vi "FPGA SPI_SPI Port.vi"(10 "Port":i8, 11 "FPGA IO":T1={"SCLK"="SCLK", "CS"="CS1", "MOSI"="MOSI", "MISO"="MISO"}) -> ()   [LabVIEW 2014]
uses:
  Controls/Port Action.ctl
  Controls/FPGA SPI_SPI Loop State.ctl
  <vilib>/Platform/TimedLoop/XDataNode/timing_clust.ctl
  <vilib>/Platform/TimedLoop/XDataNode/nitl_modes.ctl
  <vilib>/Platform/TimedLoop/XDataNode/wakeup.ctl
  <vilib>/rvi/Emulation/niFpgaGetClockAttributes.vi
  <vilib>/rvi/Emulation/niFpgaSctlEmulationGetInTimedLoop.vi
  <vilib>/rvi/Emulation/niFpgaEmulationReportErrorSimple.vi
  FPGA SPI_Globals.vi
  <vilib>/rvi/Emulation/niFpgaProcessEmulError.vi
  <vilib>/rvi/Emulation/niFpgaEmulationIsFPGAContextNoSignature.vi
  <vilib>/rvi/errors/niFpgaSetErrorForExecOnDevCompSimple.vi
  <vilib>/rvi/eio/common/nirviEmuReportErrorAndStop.vi
  <vilib>/rvi/DataTransferAndStorage/Container/Common/niFpgaContainerGetUniqueNameForEmu.vi
  <vilib>/rvi/FIFO/Fifo_Resource/nirvififoEmulationSetSize.vi
  <vilib>/rvi/FIFO/Fifo_Resource/nirviFifoEmulationQueueMgr.vi
  <instcachedir>/0/nirviFifoEmulationQueueMgr_E5CAEC123FF24DC58D834DCA3CDAA9B5.lvgen/nirviFifoEmulationQueueMgr_E5CAEC123FF24DC58D834DCA3CDAA9B5_001.vi
  <vilib>/rvi/FIFO/Fifo_Resource/nirvififoEmulationCreateLock.vi
  <vilib>/rvi/FIFO/Fifo_Resource/nirvififoEmulationObtainLock.vi
  <vilib>/rvi/FIFO/Fifo_Resource/nirvififoEmulationReleaseLock.vi
  <vilib>/rvi/occurrence/nirviWaitOnOccurrenceBase.vi
  <vilib>/rvi/errors/nirviReportUnexpectedCaseInternalError.vi
  <vilib>/rvi/errors/nirviReportUnexpectedCaseInternalError (U32).vi
  <vilib>/rvi/FIFO/Fifo_Resource/nirvififoEmulationDetermineInputValidOut.vi
  <vilib>/rvi/Emulation/niFpgaCriticalErrorInLSC.vi
  <vilib>/rvi/eio/common/nirviEmuTemplateMethod_errors.vi
  <vilib>/rvi/DataTransferAndStorage/Container/Common/niFpgaContainerSetEmuInfo.vi
  <vilib>/rvi/DataTransferAndStorage/Container/XNode/niFpgaContainer.xnode
  <vilib>/rvi/FIFO/Fifo_Resource/nirvififoEmulationRead.vi
  <vilib>/rvi/FIFO/Fifo_Resource/nirvififoEmulationWrite.vi
  <vilib>/Platform/TimedLoop/XDataNode/XDataNode.xnode
  <vilib>/eio/EIONode/EIONode.xnode
  <vilib>/rvi/LocalResourceManager/LocalResourceManager.xnode
  <vilib>/Platform/TimedLoop/XDataNode/XDNodeRunTimeDep.lvlib
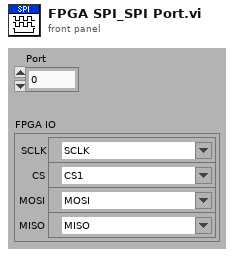
[diagram p1: front panel]
types:
  T1 = cluster{"SCLK":refnum<k21>, "CS":refnum<k21>, "MOSI":refnum<k21>, "MISO":refnum<k21>}
  T2 = cluster{"CS":u8, "CS Active State":bool, "CPOL":bool, "CPHA":bool, "Wait Ticks":u32}
  T3 = typedef "Port Action.ctl" = enum8{"Idle", "Start", "Configure Hardware", "Start Hardware", "Set Done", "Wait Until Done"}
  T4 = typedef "FPGA SPI_SPI Loop State.ctl" = enum8{"Initialize", "Read From FIFO", "Set CS", "Wait Before Set", "Set Clock", "Wait Before Reset", "Reset Clock", "Write to FIFO", "Reset CS"}
  T5 = typedef "XDNodeRunTimeDep.lvlib/timing_clust.ctl" = cluster{"Expected End [f-1]":u64, "Actual End [f-1]":u64, "Finished Late? [f-1]":bool, "Expected End [i-1]":u64, "Actual End [i-1]":u64, "Finished Late? [i-1]":bool, "Expected Start [i]":u64, "Actual Start [i]":u64, "Expected Start [f]":u64, "Actual Start [f]":u64, "Source Name":string, "Structure Name":string, "Period":i64, "Deadline":i64, "Offset":i64, "Start":i64, "Priority":i32, "Timeout":i32, "Mode":T6, "Wakeup Reason":T7, "Error":errorcluster, "Source Type":string, "Secondary Source Type":string, "Global End Time":u64, "Global Start Time":u64, "Frame Duration":u64, "Iteration Duration":u64, "Assigned CPU":i32, "I/O Scan Engine Mode":u32}
  T6 = typedef "XDNodeRunTimeDep.lvlib/nitl_modes.ctl" = enum32{"No Change", "Process missed periods, maintain original phase", "Discard missed periods, maintain original phase", "Process missed periods, ignore original phase", "Discard missed periods, ignore original phase"}
  T7 = typedef "XDNodeRunTimeDep.lvlib/wakeup.ctl" = enum32{"Normal", "Aborted", "Asynchronous wakeup", "Timing source error", "Timed loop error", "Timeout"}
  T8 = typedef "FPGA SPI_FPGA SPI State.ctl" = enum8{"Idle", "Read/Write SPI", "Configure"}
  T9 = cluster{"MOSI":bool[], "MISO":bool[], "MOSI Byte Index":i8, "MISO Byte Index":i8}
  T10 = cluster{"Next State":T4, "Wait Count":u32, "Total Bits":u16, "Current Bit":u16, "Total Bytes":u16}
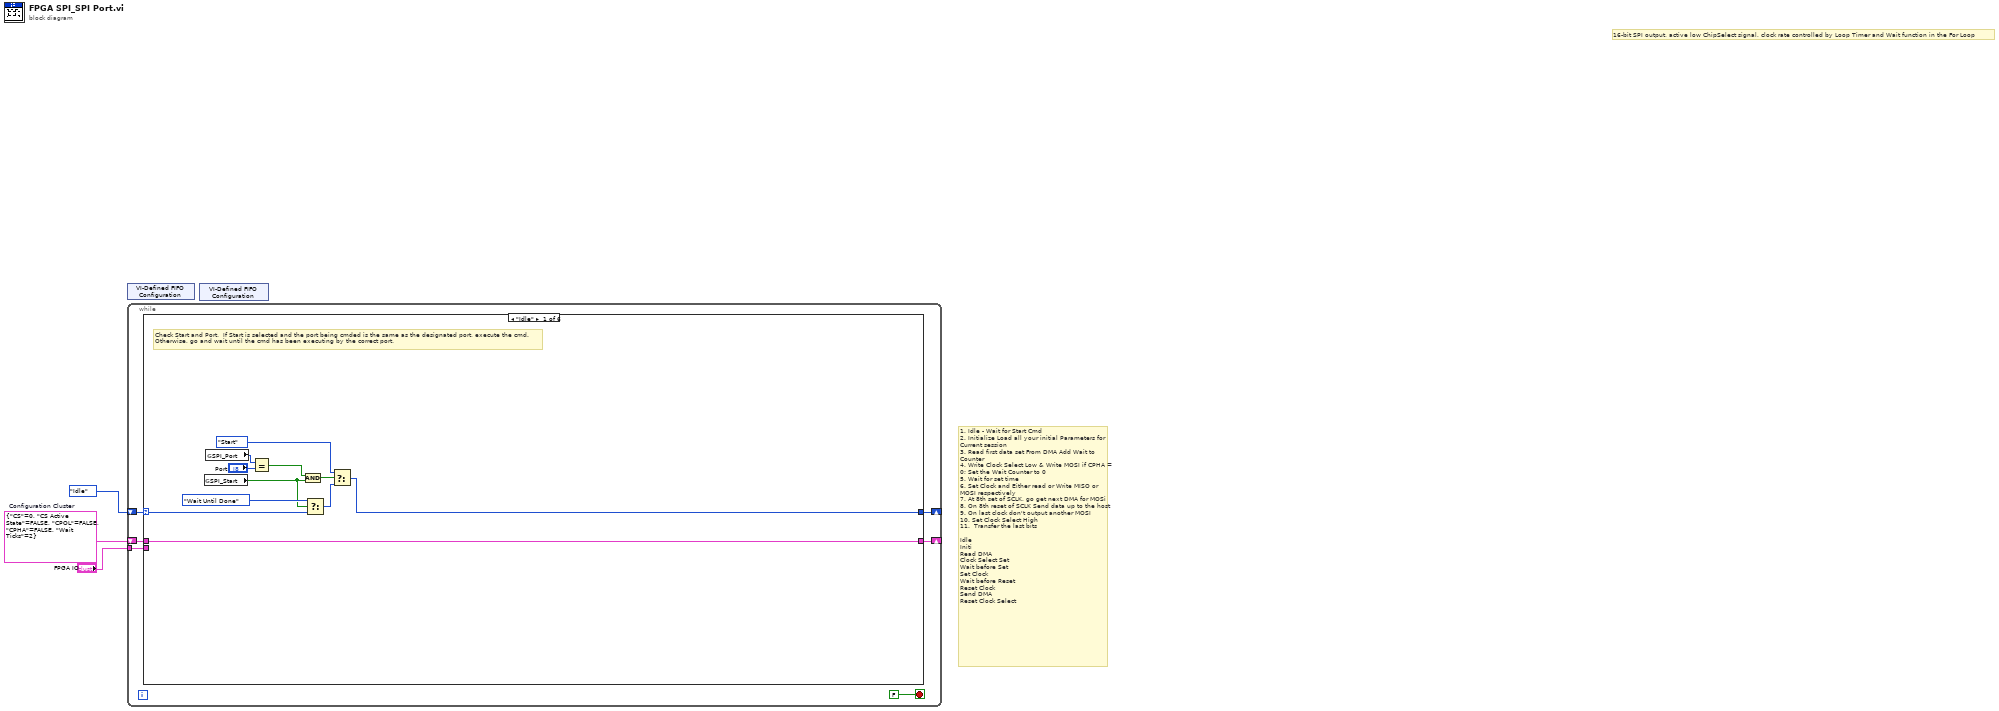
[diagram p0: block diagram]
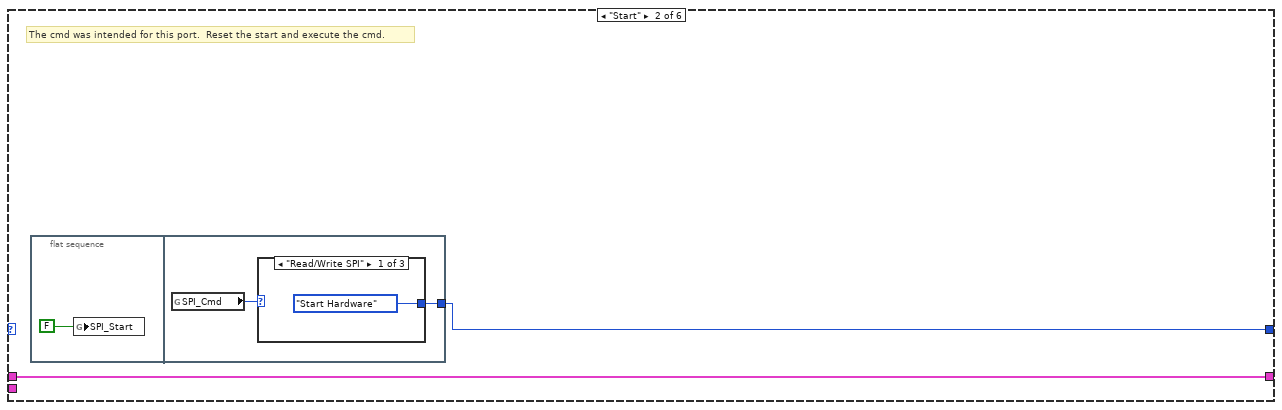
[diagram p2: hidden frame]
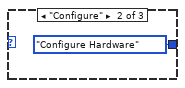
[diagram p3: hidden frame]
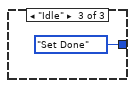
[diagram p4: hidden frame]
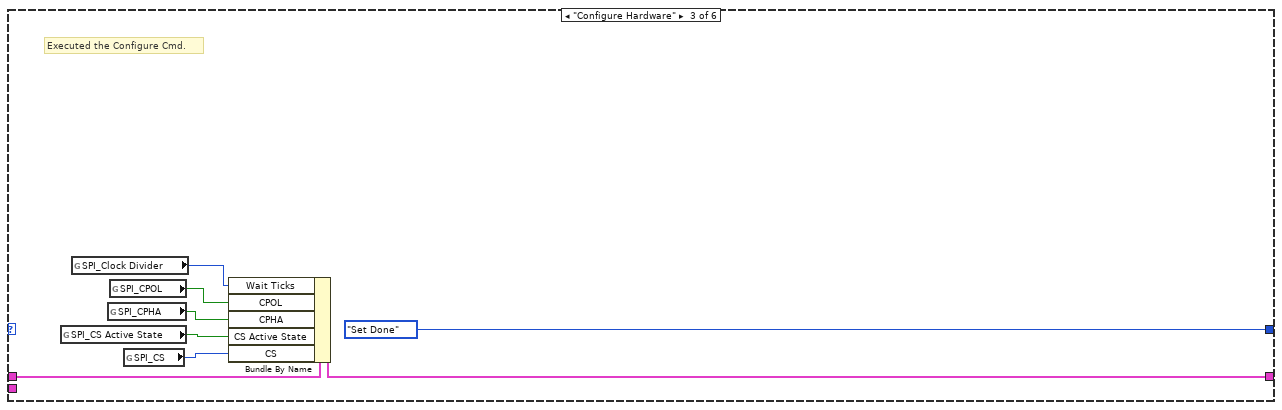
[diagram p5: hidden frame]
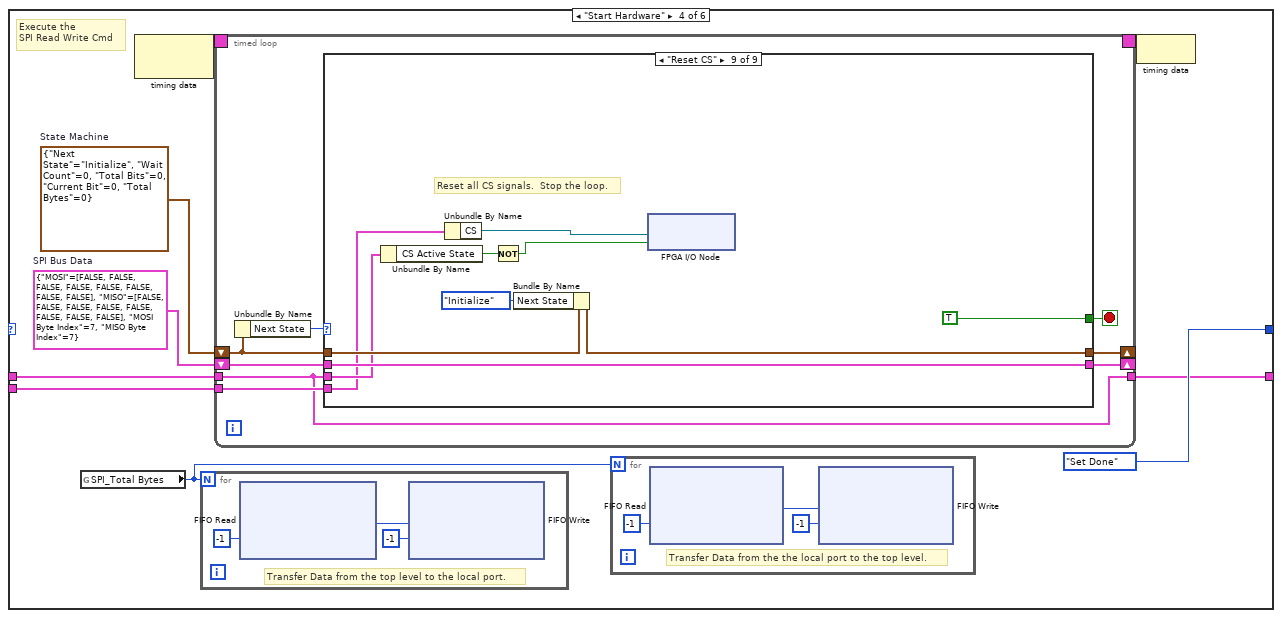
[diagram p6: hidden frame]
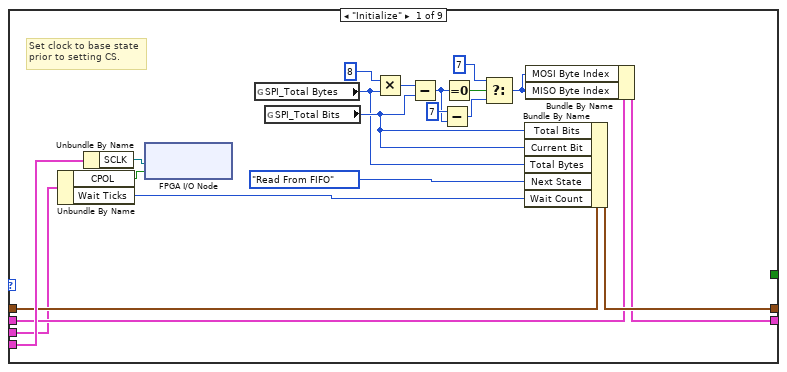
[diagram p7: hidden frame]
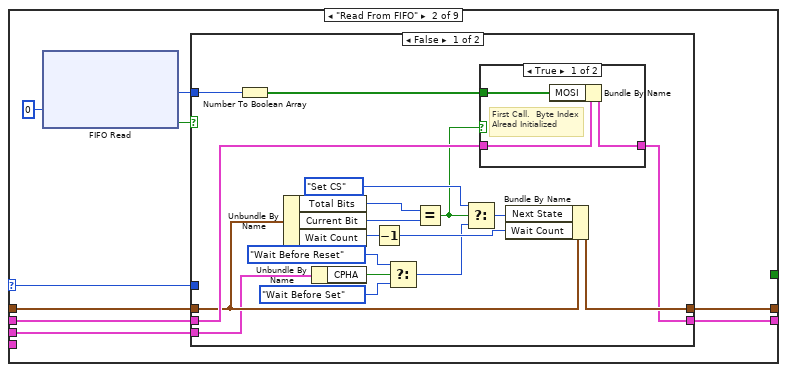
[diagram p8: hidden frame]
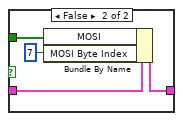
[diagram p9: hidden frame]
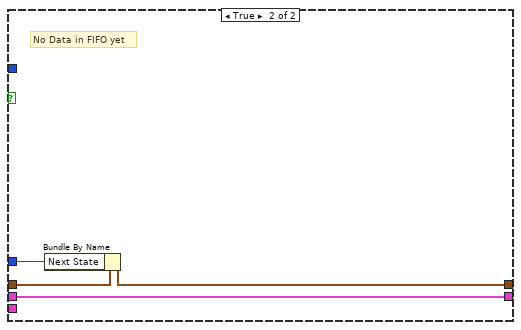
[diagram p10: hidden frame]
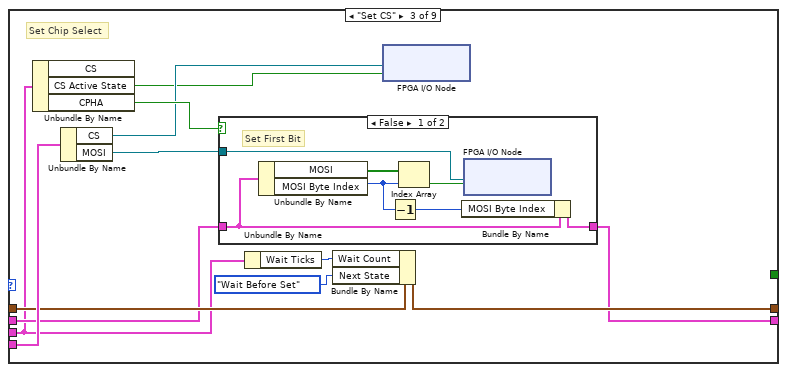
[diagram p11: hidden frame]
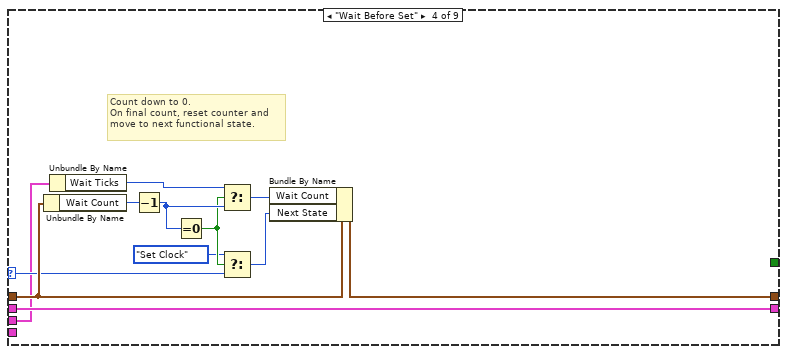
[diagram p13: hidden frame]
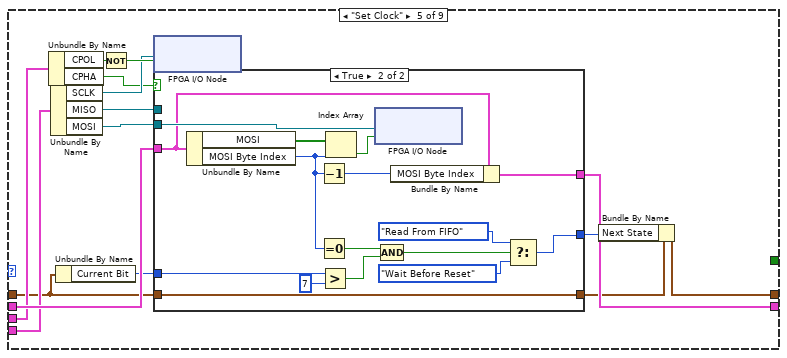
[diagram p14: hidden frame]
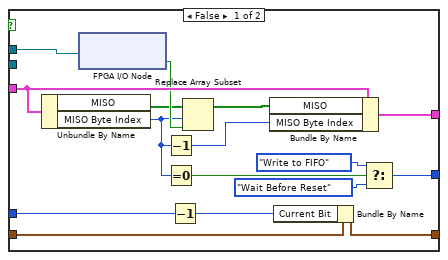
[diagram p15: hidden frame]
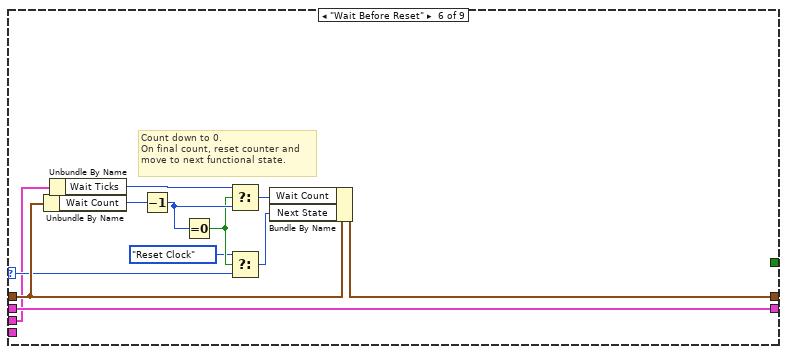
[diagram p16: hidden frame]
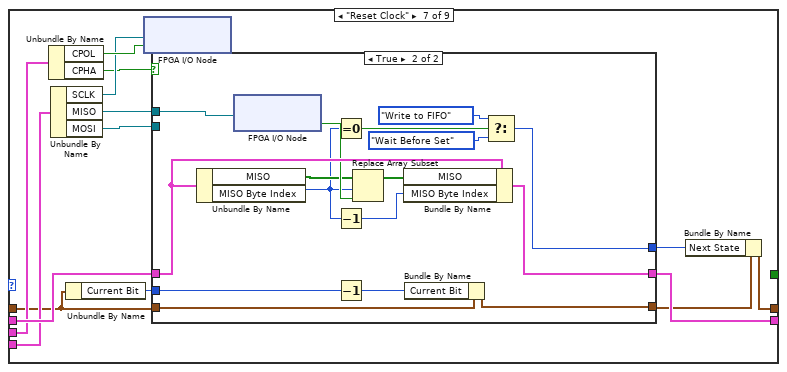
[diagram p17: hidden frame]
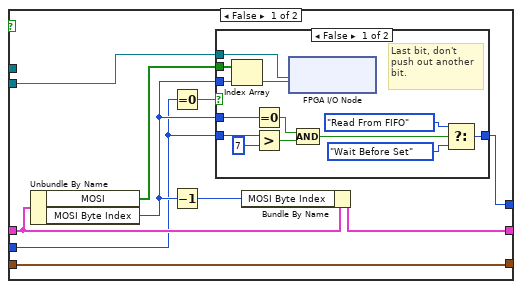
[diagram p18: hidden frame]
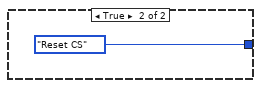
[diagram p19: hidden frame]
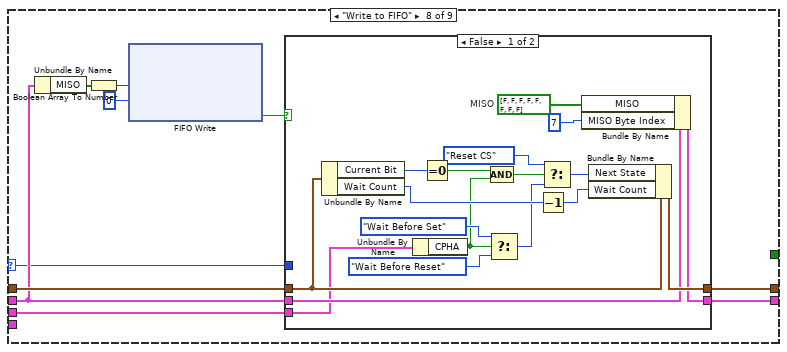
[diagram p20: hidden frame]
diagram:
  w2 = T2 {"CS"=0, "CS Active State"=FALSE, "CPOL"=FALSE, "CPHA"=FALSE, "Wait Ticks"=2}  # Configuration Cluster
  # "16-bit SPI output, active low ChipSelect signal, clock rate controlled by Loop Timer and Wait function in the For Loop"
  # "1. Idle - Wait for Start Cmd\n2. Initialize Load all your initial Parameters for Current session\n3. Read first data set From DMA Add Wait to Counter\n4. Write Clock Select Low & Write MOSI if CPHA = 0; Set the Wait Counter to 0\n5. Wait for set time\n6. Set Clock and Either read or Write MISO or MOSI respectively\n7. At 8th set of SCLK, go get next DMA for MOSi\n8. On 8th reset of SCLK Send data up to the host\n9. On last clock don't output another MOSI\n10. Set Clock Select High \n11.  Transfer the last bits\n\nIdle\nIniti\nRead DMA\nClock Select Set\nWait before Set\nSet Clock\nWait before Reset\nReset Clock\nSend DMA\nReset Clock Select"
  n1 = xnode "VI-Defined FIFO Configuration"() -> ()  [unwired: 1 out]
  n2 = while {
    shift-right: [w8] -> _
    shift-left: Port_Action."Idle" ("Action") -> [w7]
    shift-right: [w4] -> _
    shift-left: w2 -> [w6]
    tunnel: "FPGA IO" -> [w5]
    stop <- FALSE stop-if-true
    n3 = case shown="\"Idle\"" w7 {
      selector: w7 -> [w10 _ _ _ _ w314]
      tunnel: [w19 w22 Port_Action."Set Done" ("Action") Port_Action."Set Done" ("Action") Port_Action."Idle" ("Action") w313] -> w8
      tunnel: w6 -> [w14 w21 w32 w37 w309 w312]
      tunnel: w5 -> [_ _ _ w42 _ _]
      tunnel: [w14 w21 w31 w38 w309 w312] -> w4
      frame "Idle" {
        # "Check Start and Port.  If Start is selected and the port being cmded is the same as the designated port, execute the cmd.\nOtherwise, go and wait until the cmd has been executing by the correct port."
        n4 = global read "FPGA SPI_Globals.vi" "SPI_Start"() -> (w11:bool)
        n5 = global read "FPGA SPI_Globals.vi" "SPI_Port"() -> (w18:i8)
        n6 = Equal?(x=w18, y="Port") -> (x = y?=w12:bool)
        n7 = And(x=w12, y=w11) -> (x .and. y?=w16:bool)
        n8 = Select(t=Port_Action."Wait Until Done" ("Action"), s=w11, f=w10) -> (s? t:f=w15:T3)
        n9 = Select(t=Port_Action."Start" ("Action"), s=w16, f=w15) -> (s? t:f=w19:T3)
      }
      frame "Start" {
        # "The cmd was intended for this port.  Reset the start and execute the cmd."
        n10 = flat-sequence {
          tunnel: [w24] -> w22
          frame #0 {
            n11 = global write "FPGA SPI_Globals.vi" "SPI_Start"(FALSE ("Write Flag")) -> ()
          }
          frame #1 {
            n12 = global read "FPGA SPI_Globals.vi" "SPI_Cmd"() -> (w25:T8)
            n13 = case shown="\"Read/Write SPI\"" w25 {
              tunnel: [Port_Action."Start Hardware" ("Action") Port_Action."Configure Hardware" ("Action") Port_Action."Set Done" ("Action")] -> w24
              frame "Read/Write SPI" {
              }
              frame "Configure" {
              }
              frame "Idle" {
              }
            }
          }
        }
      }
      frame "Configure Hardware" {
        # "Executed the Configure Cmd."
        n14 = global read "FPGA SPI_Globals.vi" "SPI_CS Active State"() -> (w34:bool)
        n15 = global read "FPGA SPI_Globals.vi" "SPI_Clock Divider"() -> (w29:u32)
        n16 = global read "FPGA SPI_Globals.vi" "SPI_CPHA"() -> (w33:bool)
        n17 = global read "FPGA SPI_Globals.vi" "SPI_CPOL"() -> (w36:bool)
        n18 = global read "FPGA SPI_Globals.vi" "SPI_CS"() -> (w35:u8)
        n19 = Bundle By Name(cluster=w32, "Wait Ticks"=w29, "CPOL"=w36, "CPHA"=w33, "CS Active State"=w34, "CS"=w35) -> (w31:T2)
      }
      frame "Start Hardware" {
        w40 = T9 {"MOSI"=[FALSE, FALSE, FALSE, FALSE, FALSE, FALSE, FALSE, FALSE], "MISO"=[FALSE, FALSE, FALSE, FALSE, FALSE, FALSE, FALSE, FALSE], "MOSI Byte Index"=7, "MISO Byte Index"=7}  # SPI Bus Data
        w41 = T10 {"Next State"=enum."Initialize", "Wait Count"=0, "Total Bits"=0, "Current Bit"=0, "Total Bytes"=0}  # State Machine
        # "Execute the \nSPI Read Write Cmd"
        n20 = global read "FPGA SPI_Globals.vi" "SPI_Total Bytes"() -> (w39:u16)
        n21 = node-c288() -> (w44:T5)  [unwired: 1 out]
        n22 = for {
          N: w39 -> [_]
          # "Transfer Data from the top level to the local port."
          n23 = xnode ("FIFO Read")("Timeout"=-1) -> ("Element"=w50:u8)  [unwired: 1 in, 2 out]
          n24 = xnode ("FIFO Write")("Element"=w50, "Timeout"=-1) -> ()  [unwired: 1 in, 2 out]
        }
        n25 = timed-loop {
          timing-out: [_] -> w43
          timing: w44 -> [_]
          shift-right: [w59] -> _
          shift-left: w41 -> [w58]
          shift-right: [w55] -> _
          shift-left: w40 -> [w56]
          tunnel: w42 -> [w53]
          tunnel: [w52] -> w38
          tunnel: w37 -> [w52]
          stop <- w54 stop-if-true
          n26 = Unbundle By Name(w58) -> ("Next State"=w57:T4)
          n27 = case shown="\"Reset CS\"" w57 {
            selector: w57 -> [_ w80 _ w142 _ w200 _ w263 _]
            tunnel: w58 -> [w76 w83 w125 w148 w152 w207 w210 w269 w303]
            tunnel: [w75 w86 w129 w149 w164 w208 w222 w270 w304] -> w59
            tunnel: w52 -> [w61 w82 w120 w139 w159 w198 w218 w267 w300]
            tunnel: w56 -> [w62 w84 w122 w140 w160 w205 w220 w266 w301]
            tunnel: [w65 w85 w121 w140 w161 w205 w219 w265 w301] -> w55
            tunnel: w53 -> [w79 _ w128 _ w158 _ w217 _ w298]
            tunnel: [_ _ _ _ _ _ _ _ TRUE ("Start Hardware")] -> w54
            frame "Initialize" {
              # "Set clock to base state\nprior to setting CS."
              n28 = Unbundle By Name(w61) -> ("CPOL"=w77:bool, "Wait Ticks"=w60:u32)
              n29 = Unbundle By Name(w79) -> ("SCLK"=w78:refnum<k21>)
              n30 = xnode "FPGA I/O Node"("I/O Item"=w77, "FPGA I/O In"=w78) -> ()  [unwired: 1 out]
              n31 = global read "FPGA SPI_Globals.vi" "SPI_Total Bytes"() -> (w63:u16)
              n32 = global read "FPGA SPI_Globals.vi" "SPI_Total Bits"() -> (w64:u16)
              n33 = Multiply(x=u16 8 ("y"), y=w63) -> (x*y=w72:u16)
              n34 = Subtract(x=w72, y=w64) -> (x-y=w69:i8)
              n35 = Subtract(x=i8 7, y=w69) -> (x-y=w67:i8)
              n36 = Equal To 0?(x=w69) -> (x = 0?=w68:bool)
              n37 = Select(t=i8 7 ("y"), s=w68, f=w67) -> (s? t:f=w66:i8)
              n38 = Bundle By Name(cluster=w76, "Total Bits"=w64, "Current Bit"=w64, "Total Bytes"=w63, "Next State"=FPGA_SPI_SPI_Loop_State."Read From FIFO", "Wait Count"=w60) -> (w75:T10)
              n39 = Bundle By Name(cluster=w62, "MOSI Byte Index"=w66, "MISO Byte Index"=w66) -> (w65:T9)
            }
            frame "Read From FIFO" {
              n40 = xnode ("FIFO Read")("Timeout"=0) -> ("Element"=w87:u8, "Timed Out?"=w81:bool)  [unwired: 1 in, 1 out]
              n41 = case shown="False" w81 {
                tunnel: w87 -> [w106 _]
                tunnel: [w105 w114] -> w86
                tunnel: [w100 w117] -> w85
                tunnel: w84 -> [w99 w117]
                tunnel: w83 -> [w97 w115]
                tunnel: w82 -> [w89 _]
                tunnel: w80 -> [_ w116]
                frame False {
                  n42 = Number To Boolean Array(number=w106) -> (Boolean array=w98:bool[])
                  n43 = Unbundle By Name(w97) -> ("Total Bits"=w102:u16, "Current Bit"=w104:u16, "Wait Count"=w96:u32)
                  n44 = Unbundle By Name(w89) -> ("CPHA"=w93:bool)
                  n45 = Decrement(x=w96) -> (x-1=w95:u32)
                  n46 = Select(t=FPGA_SPI_SPI_Loop_State."Wait Before Reset" ("Next State"), s=w93, f=FPGA_SPI_SPI_Loop_State."Wait Before Set" ("Next State")) -> (s? t:f=w90:T4)
                  n47 = Equal?(x=w102, y=w104) -> (x = y?=w94:bool)
                  n48 = Select(t=FPGA_SPI_SPI_Loop_State."Set CS" ("Next State"), s=w94, f=w90) -> (s? t:f=w101:T4)
                  n49 = case shown="True" w94 {
                    tunnel: [w109 w113] -> w100
                    tunnel: w99 -> [w108 w112]
                    tunnel: w98 -> [w107 w111]
                    frame True {
                      # "First Call.  Byte Index Alread Initialized"
                      n50 = Bundle By Name(cluster=w108, "MOSI"=w107) -> (w109:T9)
                    }
                    frame False {
                      n51 = Bundle By Name(cluster=w112, "MOSI"=w111, "MOSI Byte Index"=i8 7) -> (w113:T9)
                    }
                  }
                  n52 = Bundle By Name(cluster=w97, "Next State"=w101, "Wait Count"=w95) -> (w105:T10)
                }
                frame True {
                  # "No Data in FIFO yet"
                  n53 = Bundle By Name(cluster=w115, "Next State"=w116) -> (w114:T10)
                }
              }
            }
            frame "Set CS" {
              # "Set Chip Select"
              n54 = Unbundle By Name(w120) -> ("CS Active State"=w118:bool, "CPHA"=w126:bool)  [unwired: 1 out]
              n55 = Unbundle By Name(w128) -> ("CS"=w119:refnum<k21>, "MOSI"=w127:refnum<k21>)
              n56 = case shown="False" w126 {
                tunnel: w122 -> [w132 w137]
                tunnel: w127 -> [w134 _]
                tunnel: [w130 w137] -> w121
                frame False {
                  # "Set First Bit"
                  n57 = Unbundle By Name(w132) -> ("MOSI"=w136:bool[], "MOSI Byte Index"=w133:i8)
                  n58 = Decrement(x=w133) -> (x-1=w131:i8)
                  n59 = Index Array(array=w136, index=w133) -> (element=w135:bool)
                  n60 = Bundle By Name(cluster=w132, "MOSI Byte Index"=w131) -> (w130:T9)
                  n61 = xnode "FPGA I/O Node"("I/O Item"=w135, "FPGA I/O In"=w134) -> ()  [unwired: 1 out]
                }
                frame True {
                }
              }
              n62 = Unbundle By Name(w120) -> ("Wait Ticks"=w124:u32)
              n63 = Bundle By Name(cluster=w125, "Wait Count"=w124, "Next State"=FPGA_SPI_SPI_Loop_State."Wait Before Set" ("Enum")) -> (w129:T10)
              n64 = xnode "FPGA I/O Node"("I/O Item"=w118, "FPGA I/O In"=w119) -> ()  [unwired: 1 out]
            }
            frame "Wait Before Set" {
              # "Count down to 0.\nOn final count, reset counter and\nmove to next functional state."
              n65 = Unbundle By Name(w148) -> ("Wait Count"=w146:u32)
              n66 = Unbundle By Name(w139) -> ("Wait Ticks"=w138:u32)
              n67 = Decrement(x=w146) -> (x-1=w147:u32)
              n68 = Equal To 0?(x=w147) -> (x = 0?=w145:bool)
              n69 = Select(t=w138, s=w145, f=w147) -> (s? t:f=w144:u32)
              n70 = Select(t=FPGA_SPI_SPI_Loop_State."Set Clock", s=w145, f=w142) -> (s? t:f=w143:T4)
              n71 = Bundle By Name(cluster=w148, "Wait Count"=w144, "Next State"=w143) -> (w149:T10)
            }
            frame "Set Clock" {
              n72 = Unbundle By Name(w159) -> ("CPOL"=w162:bool, "CPHA"=w154:bool)
              n73 = Unbundle By Name(w158) -> ("SCLK"=w155:refnum<k21>, "MISO"=w156:refnum<k21>, "MOSI"=w157:refnum<k21>)
              n74 = Unbundle By Name(w152) -> ("Current Bit"=w151:u16)
              n75 = Not(x=w162) -> (.not. x?=w163:bool)
              n76 = xnode "FPGA I/O Node"("I/O Item"=w163, "FPGA I/O In"=w155) -> ()  [unwired: 1 out]
              n77 = case shown="True" w154 {
                tunnel: [w180 w183] -> w161
                tunnel: w160 -> [w179 w184]
                tunnel: w157 -> [_ w194]
                tunnel: w156 -> [w174 _]
                tunnel: w152 -> [w173 w193]
                tunnel: [w172 w193] -> w153
                tunnel: w151 -> [w171 w191]
                tunnel: [w166 w185] -> w150
                frame False {
                  n78 = Unbundle By Name(w179) -> ("MISO"=w177:bool[], "MISO Byte Index"=w170:i8)
                  n79 = xnode "FPGA I/O Node"("FPGA I/O In"=w174) -> ("I/O Item"=w178:bool)  [unwired: 1 out]
                  n80 = Decrement(x=w170) -> (x-1=w175:i8)
                  n81 = Equal To 0?(x=w170) -> (x = 0?=w165:bool)
                  n82 = Decrement(x=w171) -> (x-1=w169:u16)
                  n83 = Replace Array Subset(array=w177, new element=w178, index=w170) -> (w176:bool[])
                  n84 = Bundle By Name(cluster=w179, "MISO"=w176, "MISO Byte Index"=w175) -> (w180:T9)
                  n85 = Bundle By Name(cluster=w173, "Current Bit"=w169) -> (w172:T10)
                  n86 = Select(t=FPGA_SPI_SPI_Loop_State."Write to FIFO" ("Enum"), s=w165, f=FPGA_SPI_SPI_Loop_State."Wait Before Reset" ("Enum")) -> (s? t:f=w166:T4)
                }
                frame True {
                  n87 = Unbundle By Name(w184) -> ("MOSI"=w196:bool[], "MOSI Byte Index"=w182:i8)
                  n88 = Decrement(x=w182) -> (x-1=w181:i8)
                  n89 = Equal To 0?(x=w182) -> (x = 0?=w192:bool)
                  n90 = Greater?(x=w191, y=u16 7 ("x")) -> (0:w189:bool)
                  n91 = Index Array(array=w196, index=w182) -> (element=w195:bool)
                  n92 = xnode "FPGA I/O Node"("I/O Item"=w195, "FPGA I/O In"=w194) -> ()  [unwired: 1 out]
                  n93 = Compound Arithmetic op=AND(w192, w189) -> (w188:bool)
                  n94 = Bundle By Name(cluster=w184, "MOSI Byte Index"=w181) -> (w183:T9)
                  n95 = Select(t=FPGA_SPI_SPI_Loop_State."Read From FIFO" ("Enum"), s=w188, f=FPGA_SPI_SPI_Loop_State."Wait Before Reset" ("Enum")) -> (s? t:f=w185:T4)
                }
              }
              n96 = Bundle By Name(cluster=w153, "Next State"=w150) -> (w164:T10)
            }
            frame "Wait Before Reset" {
              # "Count down to 0.\nOn final count, reset counter and\nmove to next functional state."
              n97 = Unbundle By Name(w207) -> ("Wait Count"=w204:u32)
              n98 = Unbundle By Name(w198) -> ("Wait Ticks"=w197:u32)
              n99 = Decrement(x=w204) -> (x-1=w206:u32)
              n100 = Equal To 0?(x=w206) -> (x = 0?=w203:bool)
              n101 = Select(t=w197, s=w203, f=w206) -> (s? t:f=w202:u32)
              n102 = Select(t=FPGA_SPI_SPI_Loop_State."Reset Clock", s=w203, f=w200) -> (s? t:f=w201:T4)
              n103 = Bundle By Name(cluster=w207, "Wait Count"=w202, "Next State"=w201) -> (w208:T10)
            }
            frame "Reset Clock" {
              n104 = Unbundle By Name(w218) -> ("CPOL"=w221:bool, "CPHA"=w213:bool)
              n105 = Unbundle By Name(w217) -> ("SCLK"=w214:refnum<k21>, "MISO"=w215:refnum<k21>, "MOSI"=w216:refnum<k21>)
              n106 = Unbundle By Name(w210) -> ("Current Bit"=w209:u16)
              n107 = xnode "FPGA I/O Node"("I/O Item"=w221, "FPGA I/O In"=w214) -> ()  [unwired: 1 out]
              n108 = case shown="True" w213 {
                tunnel: [w227 w258] -> w219
                tunnel: w220 -> [w228 w262]
                tunnel: w216 -> [w232 _]
                tunnel: w215 -> [_ w259]
                tunnel: w210 -> [w229 w256]
                tunnel: [w229 w255] -> w212
                tunnel: [w223 w249] -> w211
                tunnel: w209 -> [w224 w247]
                frame False {
                  n109 = Unbundle By Name(w228) -> ("MOSI"=w231:bool[], "MOSI Byte Index"=w225:i8)
                  n110 = Equal To 0?(x=w224) -> (x = 0?=w230:bool)
                  n111 = Decrement(x=w225) -> (x-1=w226:i8)
                  n112 = case shown="False" w230 {
                    tunnel: w232 -> [w244 _]
                    tunnel: w231 -> [w243 _]
                    tunnel: w225 -> [w242 _]
                    tunnel: w225 -> [w238 _]
                    tunnel: w224 -> [w237 _]
                    tunnel: [w233 FPGA_SPI_SPI_Loop_State."Reset CS" ("Enum")] -> w223
                    frame False {
                      # "Last bit, don't\npush out another\nbit."
                      n113 = Index Array(array=w243, index=w242) -> (element=w245:bool)
                      n114 = Equal To 0?(x=w238) -> (x = 0?=w240:bool)
                      n115 = Greater?(x=w237, y=u16 7 ("x")) -> (0:w241:bool)
                      n116 = xnode "FPGA I/O Node"("I/O Item"=w245, "FPGA I/O In"=w244) -> ()  [unwired: 1 out]
                      n117 = Compound Arithmetic op=AND(w240, w241) -> (w234:bool)
                      n118 = Select(t=FPGA_SPI_SPI_Loop_State."Read From FIFO" ("Enum"), s=w234, f=FPGA_SPI_SPI_Loop_State."Wait Before Set" ("Enum")) -> (s? t:f=w233:T4)
                    }
                    frame True {
                    }
                  }
                  n119 = Bundle By Name(cluster=w228, "MOSI Byte Index"=w226) -> (w227:T9)
                }
                frame True {
                  n120 = Unbundle By Name(w262) -> ("MISO"=w260:bool[], "MISO Byte Index"=w251:i8)
                  n121 = xnode "FPGA I/O Node"("FPGA I/O In"=w259) -> ("I/O Item"=w261:bool)  [unwired: 1 out]
                  n122 = Equal To 0?(x=w251) -> (x = 0?=w248:bool)
                  n123 = Decrement(x=w251) -> (x-1=w254:i8)
                  n124 = Decrement(x=w247) -> (x-1=w250:u16)
                  n125 = Replace Array Subset(array=w260, new element=w261, index=w251) -> (w257:bool[])
                  n126 = Bundle By Name(cluster=w262, "MISO"=w257, "MISO Byte Index"=w254) -> (w258:T9)
                  n127 = Bundle By Name(cluster=w256, "Current Bit"=w250) -> (w255:T10)
                  n128 = Select(t=FPGA_SPI_SPI_Loop_State."Write to FIFO" ("Enum"), s=w248, f=FPGA_SPI_SPI_Loop_State."Wait Before Set" ("Enum")) -> (s? t:f=w249:T4)
                }
              }
              n129 = Bundle By Name(cluster=w212, "Next State"=w211) -> (w222:T10)
            }
            frame "Write to FIFO" {
              n130 = Unbundle By Name(w266) -> ("MISO"=w272:bool[])
              n131 = Boolean Array To Number(Boolean array=w272) -> (number=w271:u8)
              n132 = xnode ("FIFO Write")("Element"=w271, "Timeout"=0) -> ("Timed Out?"=w264:bool)  [unwired: 1 in, 1 out]
              n133 = case shown="False" w264 {
                tunnel: [w290 w292] -> w270
                tunnel: w269 -> [w289 w293]
                tunnel: w267 -> [w273 _]
                tunnel: w266 -> [w276 w294]
                tunnel: [w274 w294] -> w265
                tunnel: w263 -> [_ w291]
                frame False {
                  w277 = bool[] [FALSE, FALSE, FALSE, FALSE, FALSE, FALSE, FALSE, FALSE]  # MISO
                  n134 = Unbundle By Name(w289) -> ("Current Bit"=w288:u16, "Wait Count"=w285:u32)
                  n135 = Unbundle By Name(w273) -> ("CPHA"=w279:bool)
                  n136 = Equal To 0?(x=w288) -> (x = 0?=w281:bool)
                  n137 = Select(t=FPGA_SPI_SPI_Loop_State."Wait Before Set" ("Next State"), s=w279, f=FPGA_SPI_SPI_Loop_State."Wait Before Reset" ("Next State")) -> (s? t:f=w282:T4)
                  n138 = Compound Arithmetic op=AND(w281, w279) -> (w280:bool)
                  n139 = Decrement(x=w285) -> (x-1=w278:u32)
                  n140 = Select(t=FPGA_SPI_SPI_Loop_State."Reset CS" ("Next State"), s=w280, f=w282) -> (s? t:f=w286:T4)
                  n141 = Bundle By Name(cluster=w276, "MISO"=w277, "MISO Byte Index"=i8 7) -> (w274:T9)
                  n142 = Bundle By Name(cluster=w289, "Next State"=w286, "Wait Count"=w278) -> (w290:T10)
                }
                frame True {
                  n143 = Bundle By Name(cluster=w293, "Next State"=w291) -> (w292:T10)
                }
              }
            }
            frame "Reset CS" {
              # "Reset all CS signals.  Stop the loop."
              n144 = Unbundle By Name(w300) -> ("CS Active State"=w299:bool)
              n145 = Unbundle By Name(w298) -> ("CS"=w297:refnum<k21>)
              n146 = Not(x=w299) -> (.not. x?=w295:bool)
              n147 = Bundle By Name(cluster=w303, "Next State"=FPGA_SPI_SPI_Loop_State."Initialize" ("Enum")) -> (w304:T10)
              n148 = xnode "FPGA I/O Node"("I/O Item"=w295, "FPGA I/O In"=w297) -> ()  [unwired: 1 out]
            }
          }
        }
        n149 = for {
          N: w39 -> [_]
          # "Transfer Data from the the local port to the top level."
          n150 = xnode ("FIFO Read")("Timeout"=-1) -> ("Element"=w47:u8)  [unwired: 1 in, 2 out]
          n151 = xnode ("FIFO Write")("Element"=w47, "Timeout"=-1) -> ()  [unwired: 1 in, 2 out]
        }
        n152 = node-c288(w43) -> ()
      }
      frame "Set Done" {
        # "Set the done flag"
        n153 = global write "FPGA SPI_Globals.vi" "SPI_Done"(TRUE ("Done")) -> ()
      }
      frame "Wait Until Done" {
        # "Wait until the executing port finishes."
        n154 = global read "FPGA SPI_Globals.vi" "SPI_Done"() -> (w316:bool)
        n155 = Select(t=Port_Action."Idle" ("Action"), s=w316, f=w314) -> (s? t:f=w313:T3)
      }
    }
  }
  n156 = xnode "VI-Defined FIFO Configuration"() -> ()  [unwired: 1 out]
